vi "CleanUp.vi"(8 "error in (no error)":errorcluster, 11 "object in":refnum<class "Modbus TCP.lvclass">) -> (0 "error out":errorcluster, 3 "object out":refnum<class "Modbus TCP.lvclass">)   [LabVIEW 2023, in "HardwareAbstractionLayer_LVOOP.lvlib" / "Modbus TCP.lvclass"]
uses:
  Modbus TCP.lvclass
  Modbus TCP.lvclass/Modbus TCP.ctl
  <vilib>/NI/Modbus Library/API/Master/Modbus Master.lvclass
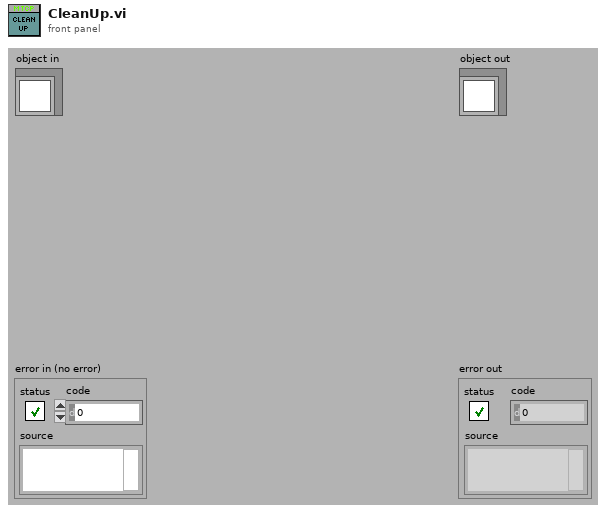
[diagram p1: front panel]
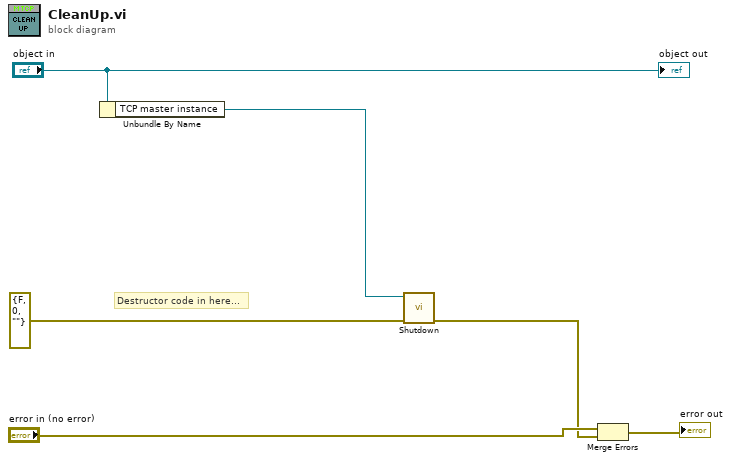
[diagram p0: block diagram]
diagram:
  # "Destructor code in here..."
  n1 = Unbundle By Name("object in") -> ("TCP master instance"=w2:refnum<class "Modbus Master.lvclass">)
  n2 = call-dynamic "Shutdown.vi"("error in"=errorcluster {"status"=FALSE, "code"=0, "source"=""} ("error in (no error)"), "Modbus master in"=w2) -> ("error out"=w1:errorcluster)  [unwired: 9 in]
  n3 = Merge Errors("error in (no error)", w1) -> (→"error out":errorcluster)
  "object out" <- "object in"
